vi "TDTSyn-Get Channel Counts.vi"(0 "Synapse URL":string, 7 "TankCode pattern":string, 11 "error in (no error)":errorcluster) -> (4 "Channel counts":i32[](array[numeric]), 15 "error out":errorcluster)   [LabVIEW 2015]
uses:
  <vilib>/regexp/Match Regular Expression.xnode
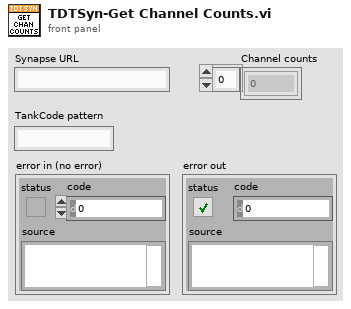
[diagram p1: front panel]
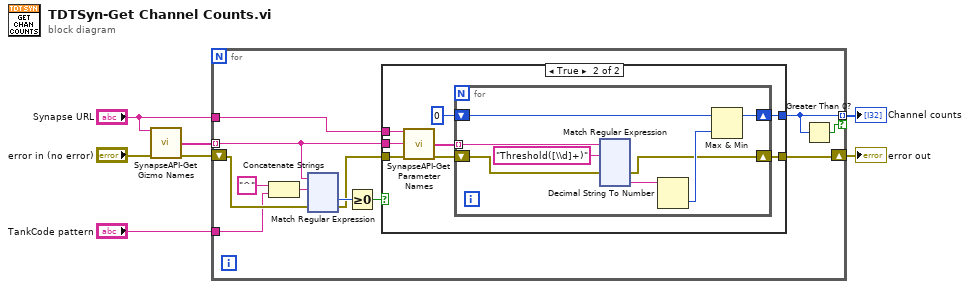
[diagram p0: block diagram]
diagram:
  n1 = call "SynapseAPI-Get Gizmo Names.vi"("URL"="Synapse URL", "error in (no error)"="error in (no error)") -> ("names"=w4:string[], "error out"=w5:errorcluster)  [unwired: 12 in]
  n2 = for {
    tunnel: w4 -> [w13] mode=indexing
    shift-right: [w12] -> w2
    shift-left: w5 -> [w18]
    tunnel: "Synapse URL" -> [w19]
    tunnel: [w10] -> w7 mode=indexing if=w11
    tunnel: "TankCode pattern" -> [w8]
    n3 = Concatenate Strings("^" ("regular expression"), w8) -> (w9:string)
    n4 = xnode "Match Regular Expression"("input string"=w13, "regular expression"=w9, "error in"=w18) -> ("offset past match"=w16:i32, "error out"=w15:errorcluster)  [unwired: 3 in, 3 out]
    n5 = Greater Or Equal To 0?(x=w16) -> (x >= 0?=w14:bool)
    n6 = case shown="True" w14 {
      tunnel: w19 -> [_ w28]
      tunnel: w15 -> [w20 w27]
      tunnel: w13 -> [_ w26]
      tunnel: [_ w22] -> w10
      tunnel: [w20 w21] -> w12
      frame False {
      }
      frame True {
        n7 = call "SynapseAPI-Get Parameter Names.vi"("URL"=w28, "gizmo"=w26, "error in (no error)"=w27) -> ("parameters"=w24:string[], "error out"=w25:errorcluster)  [unwired: 11 in]
        n8 = for {
          shift-right: [w30] -> w21
          shift-left: w25 -> [w35]
          tunnel: w24 -> [w36] mode=indexing
          shift-right: [w33] -> w22
          shift-left: 0 -> [w32]
          n9 = xnode "Match Regular Expression"("input string"=w36, "regular expression"="Threshold([\\d]+)", "error in"=w35) -> ("error out"=w30:errorcluster, "submatch 1"=w29:string)  [unwired: 3 in, 4 out]
          n10 = Decimal String To Number(string=w29) -> (number=w31:i32)  [unwired: 2 in, 1 out]
          n11 = Max & Min(x=w32, y=w31) -> (max(x,y)=w33:i32)  [unwired: 1 out]
        }
      }
    }
    n12 = Greater Than 0?(x=w10) -> (x > 0?=w11:bool)
  }
  "Channel counts" <- w7
  "error out" <- w2
